vi "dual_priority_encoder.vi"() -> ()   [LabVIEW 2019]
panel:
  in  "En":bool
  out "BVALID":bool
  out "B0":bool
  out "B1":bool
  out "B2":bool
  out "AVALID":bool
  out "A0":bool
  out "A1":bool
  out "A2":bool
  in  "i 0":bool
  in  "i1":bool
  in  "?":bool
  in  "?":bool
  in  "i4":bool
  in  "i5":bool
  in  "i6":bool
  in  "i7":bool
  # "1ST HIGHEST PRIORITY OUT"
  # "DUAL PRIORITY ENCODER"
  # "2ND HIGHEST PRIORITY OUT"
  # "i3"
  # "i2"
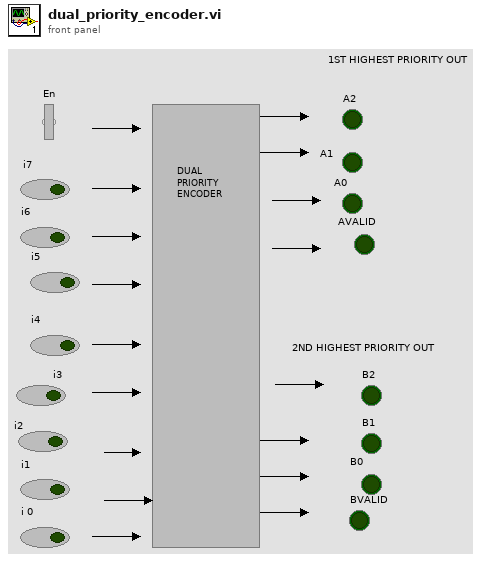
[diagram p1: front panel]
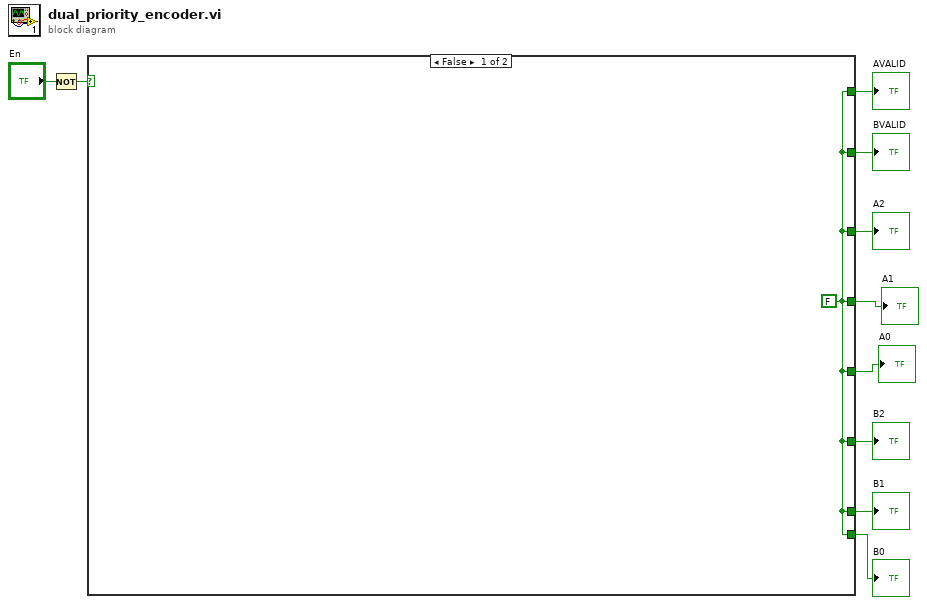
[diagram p0: block diagram]
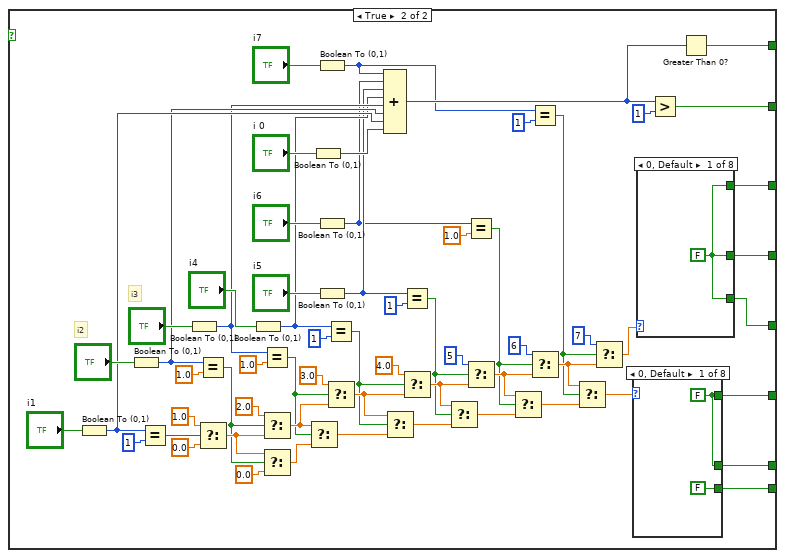
[diagram p2: hidden frame]
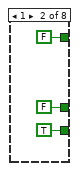
[diagram p3: hidden frame]
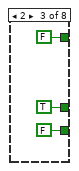
[diagram p4: hidden frame]
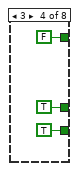
[diagram p5: hidden frame]
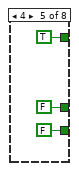
[diagram p6: hidden frame]
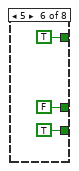
[diagram p7: hidden frame]
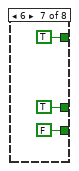
[diagram p8: hidden frame]
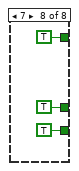
[diagram p9: hidden frame]
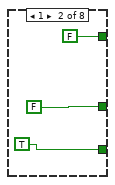
[diagram p10: hidden frame]
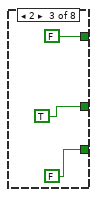
[diagram p11: hidden frame]
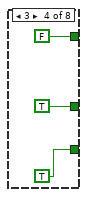
[diagram p12: hidden frame]
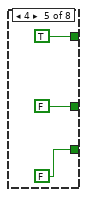
[diagram p13: hidden frame]
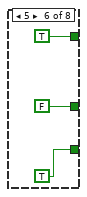
[diagram p14: hidden frame]
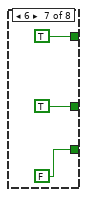
[diagram p15: hidden frame]
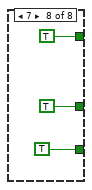
[diagram p16: hidden frame]
diagram:
  n1 = Not(x="En") -> (.not. x?=w3:bool)
  n2 = case shown="False" w3 {
    tunnel: [w11 w63] -> w9
    tunnel: [w11 w62] -> w2
    tunnel: [w11 w61] -> w1
    tunnel: [w11 w60] -> w8
    tunnel: [w11 w59] -> w7
    tunnel: [w11 w58] -> w6
    tunnel: [w11 w47] -> w5
    tunnel: [w11 w46] -> w4
    frame False {
      w11 = FALSE
    }
    frame True {
      # "i3"
      # "i2"
      n3 = Boolean To (0,1)(Boolean="i1") -> (0, 1=w37:i16)
      n4 = Boolean To (0,1)(Boolean="?") -> (0, 1=w36:i16)
      n5 = Equal?(x=w37, y=i16 1) -> (x = y?=w38:bool)
      n6 = Boolean To (0,1)(Boolean="?") -> (0, 1=w35:i16)
      n7 = Equal?(x=w36, y=1.0) -> (x = y?=w27:bool)
      n8 = Select(t=1.0, s=w38, f=0.0) -> (s? t:f=w28:dbl)
      n9 = Boolean To (0,1)(Boolean="i4") -> (0, 1=w34:i16)
      n10 = Equal?(x=w35, y=1.0) -> (x = y?=w25:bool)
      n11 = Select(t=2.0, s=w27, f=w28) -> (s? t:f=w26:dbl)
      n12 = Select(t=w28, s=w27, f=0.0) -> (s? t:f=w14:dbl)
      n13 = Select(t=w26, s=w25, f=w14) -> (s? t:f=w23:dbl)
      n14 = Boolean To (0,1)(Boolean="i 0") -> (0, 1=w49:i16)
      n15 = Boolean To (0,1)(Boolean="i7") -> (0, 1=w31:i16)
      n16 = Boolean To (0,1)(Boolean="i6") -> (0, 1=w32:i16)
      n17 = Boolean To (0,1)(Boolean="i5") -> (0, 1=w33:i16)
      n18 = Equal?(x=w34, y=i16 1) -> (x = y?=w22:bool)
      n19 = Select(t=3.0, s=w25, f=w26) -> (s? t:f=w24:dbl)
      n20 = Compound Arithmetic op=ADD(w31, w32, w33, w34, w35, w36, w37, w49) -> (w48:i16)
      n21 = Select(t=w24, s=w22, f=w23) -> (s? t:f=w20:dbl)
      n22 = Equal?(x=w33, y=i16 1) -> (x = y?=w19:bool)
      n23 = Select(t=4.0, s=w22, f=w24) -> (s? t:f=w21:dbl)
      n24 = Select(t=w21, s=w19, f=w20) -> (s? t:f=w17:dbl)
      n25 = Equal?(x=w32, y=1.0) -> (x = y?=w15:bool)
      n26 = Select(t=5, s=w19, f=w21) -> (s? t:f=w18:dbl)
      n27 = Select(t=w18, s=w15, f=w17) -> (s? t:f=w16:dbl)
      n28 = Equal?(x=w31, y=1) -> (x = y?=w13:bool)
      n29 = Select(t=6, s=w15, f=w18) -> (s? t:f=w29:dbl)
      n30 = Select(t=w29, s=w13, f=w16) -> (s? t:f=w12:dbl)
      n31 = Select(t=7, s=w13, f=w29) -> (s? t:f=w30:dbl)
      n32 = case shown="0, Default" w12 {
        tunnel: [w75 FALSE FALSE FALSE TRUE TRUE TRUE TRUE] -> w60
        tunnel: [w75 FALSE TRUE TRUE FALSE FALSE TRUE TRUE] -> w59
        tunnel: [FALSE TRUE FALSE TRUE FALSE TRUE FALSE TRUE] -> w58
        frame 0, Default {
          w75 = FALSE
        }
        frame 1 {
        }
        frame 2 {
        }
        frame 3 {
        }
        frame 4 {
        }
        frame 5 {
        }
        frame 6 {
        }
        frame 7 {
        }
      }
      n33 = case shown="0, Default" w30 {
        tunnel: [w97 FALSE FALSE FALSE TRUE TRUE TRUE TRUE] -> w63
        tunnel: [w97 TRUE FALSE TRUE FALSE TRUE FALSE TRUE] -> w62
        tunnel: [w97 FALSE TRUE TRUE FALSE FALSE TRUE TRUE] -> w61
        frame 0, Default {
          w97 = FALSE
        }
        frame 1 {
        }
        frame 2 {
        }
        frame 3 {
        }
        frame 4 {
        }
        frame 5 {
        }
        frame 6 {
        }
        frame 7 {
        }
      }
      n34 = Greater?(x=w48, y=1) -> (0:w46:bool)
      n35 = Greater Than 0?(x=w48) -> (x > 0?=w47:bool)
    }
  }
  "A2" <- w9
  "A1" <- w1
  "A0" <- w2
  "B2" <- w8
  "B1" <- w7
  "B0" <- w6
  "AVALID" <- w5
  "BVALID" <- w4
